vi "Odor_Control_m.vi"() -> ()   [LabVIEW 2014]
uses:
  <vilib>/Utility/file.llb/Read From Spreadsheet File (DBL).vi
  <vilib>/Utility/file.llb/Read From Spreadsheet File (I64).vi
  Image Aquisition - Labview/Image Recorder/experiment state global.vi
  <vilib>/Utility/file.llb/Write To Spreadsheet File (string).vi
panel:
  in  "File with probe valve sequence":path=path "\\\\LABNAS40\\Luis/2016/Physiology_Odor_Responses/Calibration_gwn/gaussian_wn.txt"
  in  "Probe valves from file?":bool
  in  "File with valve sequence":path=path "\\\\LABNAS40\\Luis/2016/Physiology_Odor_Responses/Calibration_gwn/gaussian_wn.txt"
  in  "Valves from file?":bool
  in  "Sync Mode":bool=TRUE
  out "Security Valve \nfor Odor 1":bool
  in  "threshold \nfor odor 1":dbl
  in  "File with signal for odor 2":path=path "\\\\LABNAS40\\Luis/2016/Physiology_Odor_Responses/PL1ol/20170213/step_log_pyramid_w_sigmoid.txt"
  in  "File with signal for odor 1":path=path "\\\\LABNAS40\\Luis/2016/Physiology_Odor_Responses/PL1ol/20170211/Log_pulse_train.txt"
  in  "ODOR 2":bool=TRUE
  in  "ODOR 1":bool
  in  "ODOR 2 FLOW %":dbl(slide) scale=0.0..100.0
  in  "ODOR 1 FLOW %":dbl(slide) scale=0.0..100.0
  in  "ODOR 2":bool=TRUE
  in  "ODOR 1":bool
  in  "TOLERANCE \nFOR CLOSING \nPROBE VALVE":dbl=0.5
  in  "MODE SELECTOR":string(combo)="MANUAL"
  out "Path":path=path "D:/Luis/2017/0212/2118"
  in  "8":bool
  in  "7":bool
  in  "6":bool
  in  "5":bool
  in  "4":bool
  in  "3":bool
  in  "2":bool
  in  "1":bool
  in  "Start Recording":bool
  in  "extra label:":string="Calibration_S3"
  in  "Save To:":path=path "D:/Luis"
  in  "CLEAR stored data":bool
  in  "Select signal to plot":T1(ring)=enum."odor 2 flow rate"
  out "XY Graph":T2(graph)
  in  "Air Flow Rate \n(L/min)":dbl
  in  "odor 2 between experiments":dbl
  in  "odor 2 signal parameters":T3={"temporal ramp type"=enum."Sine", "period(s)"=20.0, "high limit"=0.0, "low limit"=0.0, "duty cycle (sq wave)"=50.0} {"low limit" format="%#_6p"}
  in  "odor 1 between experiments":dbl
  in  "Sync Signal To \nImage Aquisition":bool=TRUE
  in  "ENABLE MFCs":bool
  in  "Restart Signal":bool
  in  "odor 1 signal parameters":T3={"temporal ramp type"=enum."Triangle", "period(s)"=20.0, "high limit"=100.0, "low limit"=10.0, "duty cycle (sq wave)"=50.0} {"low limit" format="%#_6p"}
  in  "update period (ms)":u32=50
  in  "?":bool
  # "NOTE: Always start with Start Recording OFF, don't turn OFF while running"
  # "Manual Stop"
  # "VALVE CONTROL"
  # "MANUAL"
  # "FROM FILE"
  # "VALVE FROM FILE CONTROL"
  # "PREDEFINED WAVEFORM"
  # "PARAMETERS FOR BACKWASH PREVENTION"
  # "Currently the security valve for \nodor 1 is not installed so be careful!"
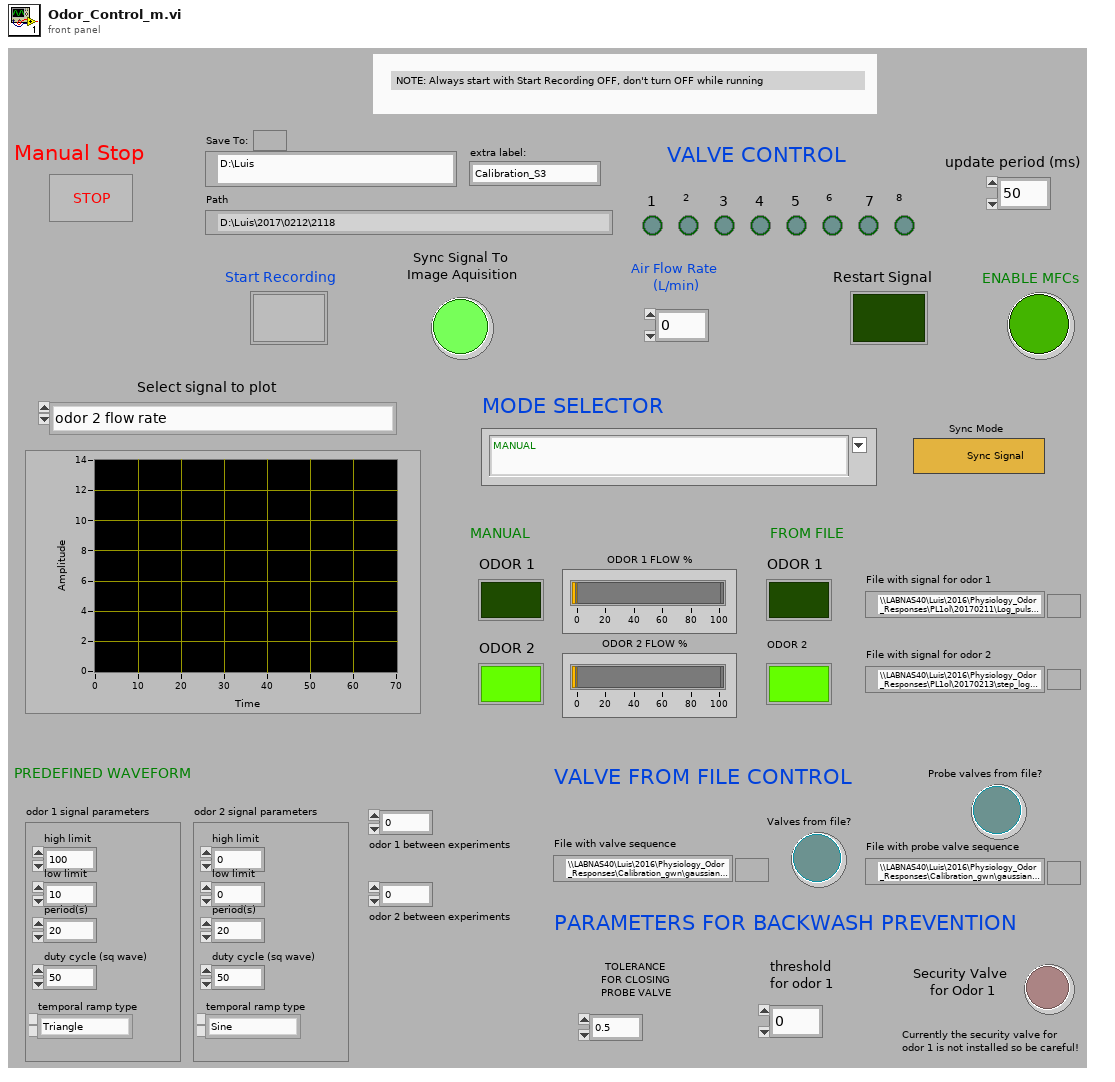
[diagram p1: front panel]
types:
  T1 = enum16{"air setpoint", "air flow rate", "odor 1 set point", "odor 1 flow rate", "odor 2 setpoint", "odor 2 flow rate", "pid reading", "led current", "led voltage", "led setpoint", "led temperature"}
  T2 = cluster{"Value Array":dbl[], "Value Array":dbl[]}
  T3 = cluster{"temporal ramp type":enum16{"Sine", "Triangle", "Sawtooth", "Square", "Exponential"}, "period(s)":dbl, "high limit":dbl, "low limit":dbl, "duty cycle (sq wave)":dbl}
  T4 = cluster{"analog output channels":cluster{"air ao":refnum<k21>, "odor 1 ao":refnum<k21>, "odor 2 ao":refnum<k21>}, "analog input channels":cluster{"air ai":refnum<k21>, "odor 1 ai":refnum<k21>, "odor 2 ai":refnum<k21>, "pid sensor 1 ai":refnum<k21>, "pid sensor 2 ai":refnum<k21>}, "digital control lines":cluster{"air close":refnum<k21>, "air purge":refnum<k21>, "odor 1 close":refnum<k21>, "odor 1 purge":refnum<k21>, "odor 2 close":refnum<k21>, "odor 2 purge":refnum<k21>}}
  T5 = enum16{"Reset Table", "Get Values", "Add Value", "Get Table", "Get Spreadsheet", "set stack writer"}
  T6 = cluster{"experiment started":bool, "experiment ended":bool, "experiment start time":u32}
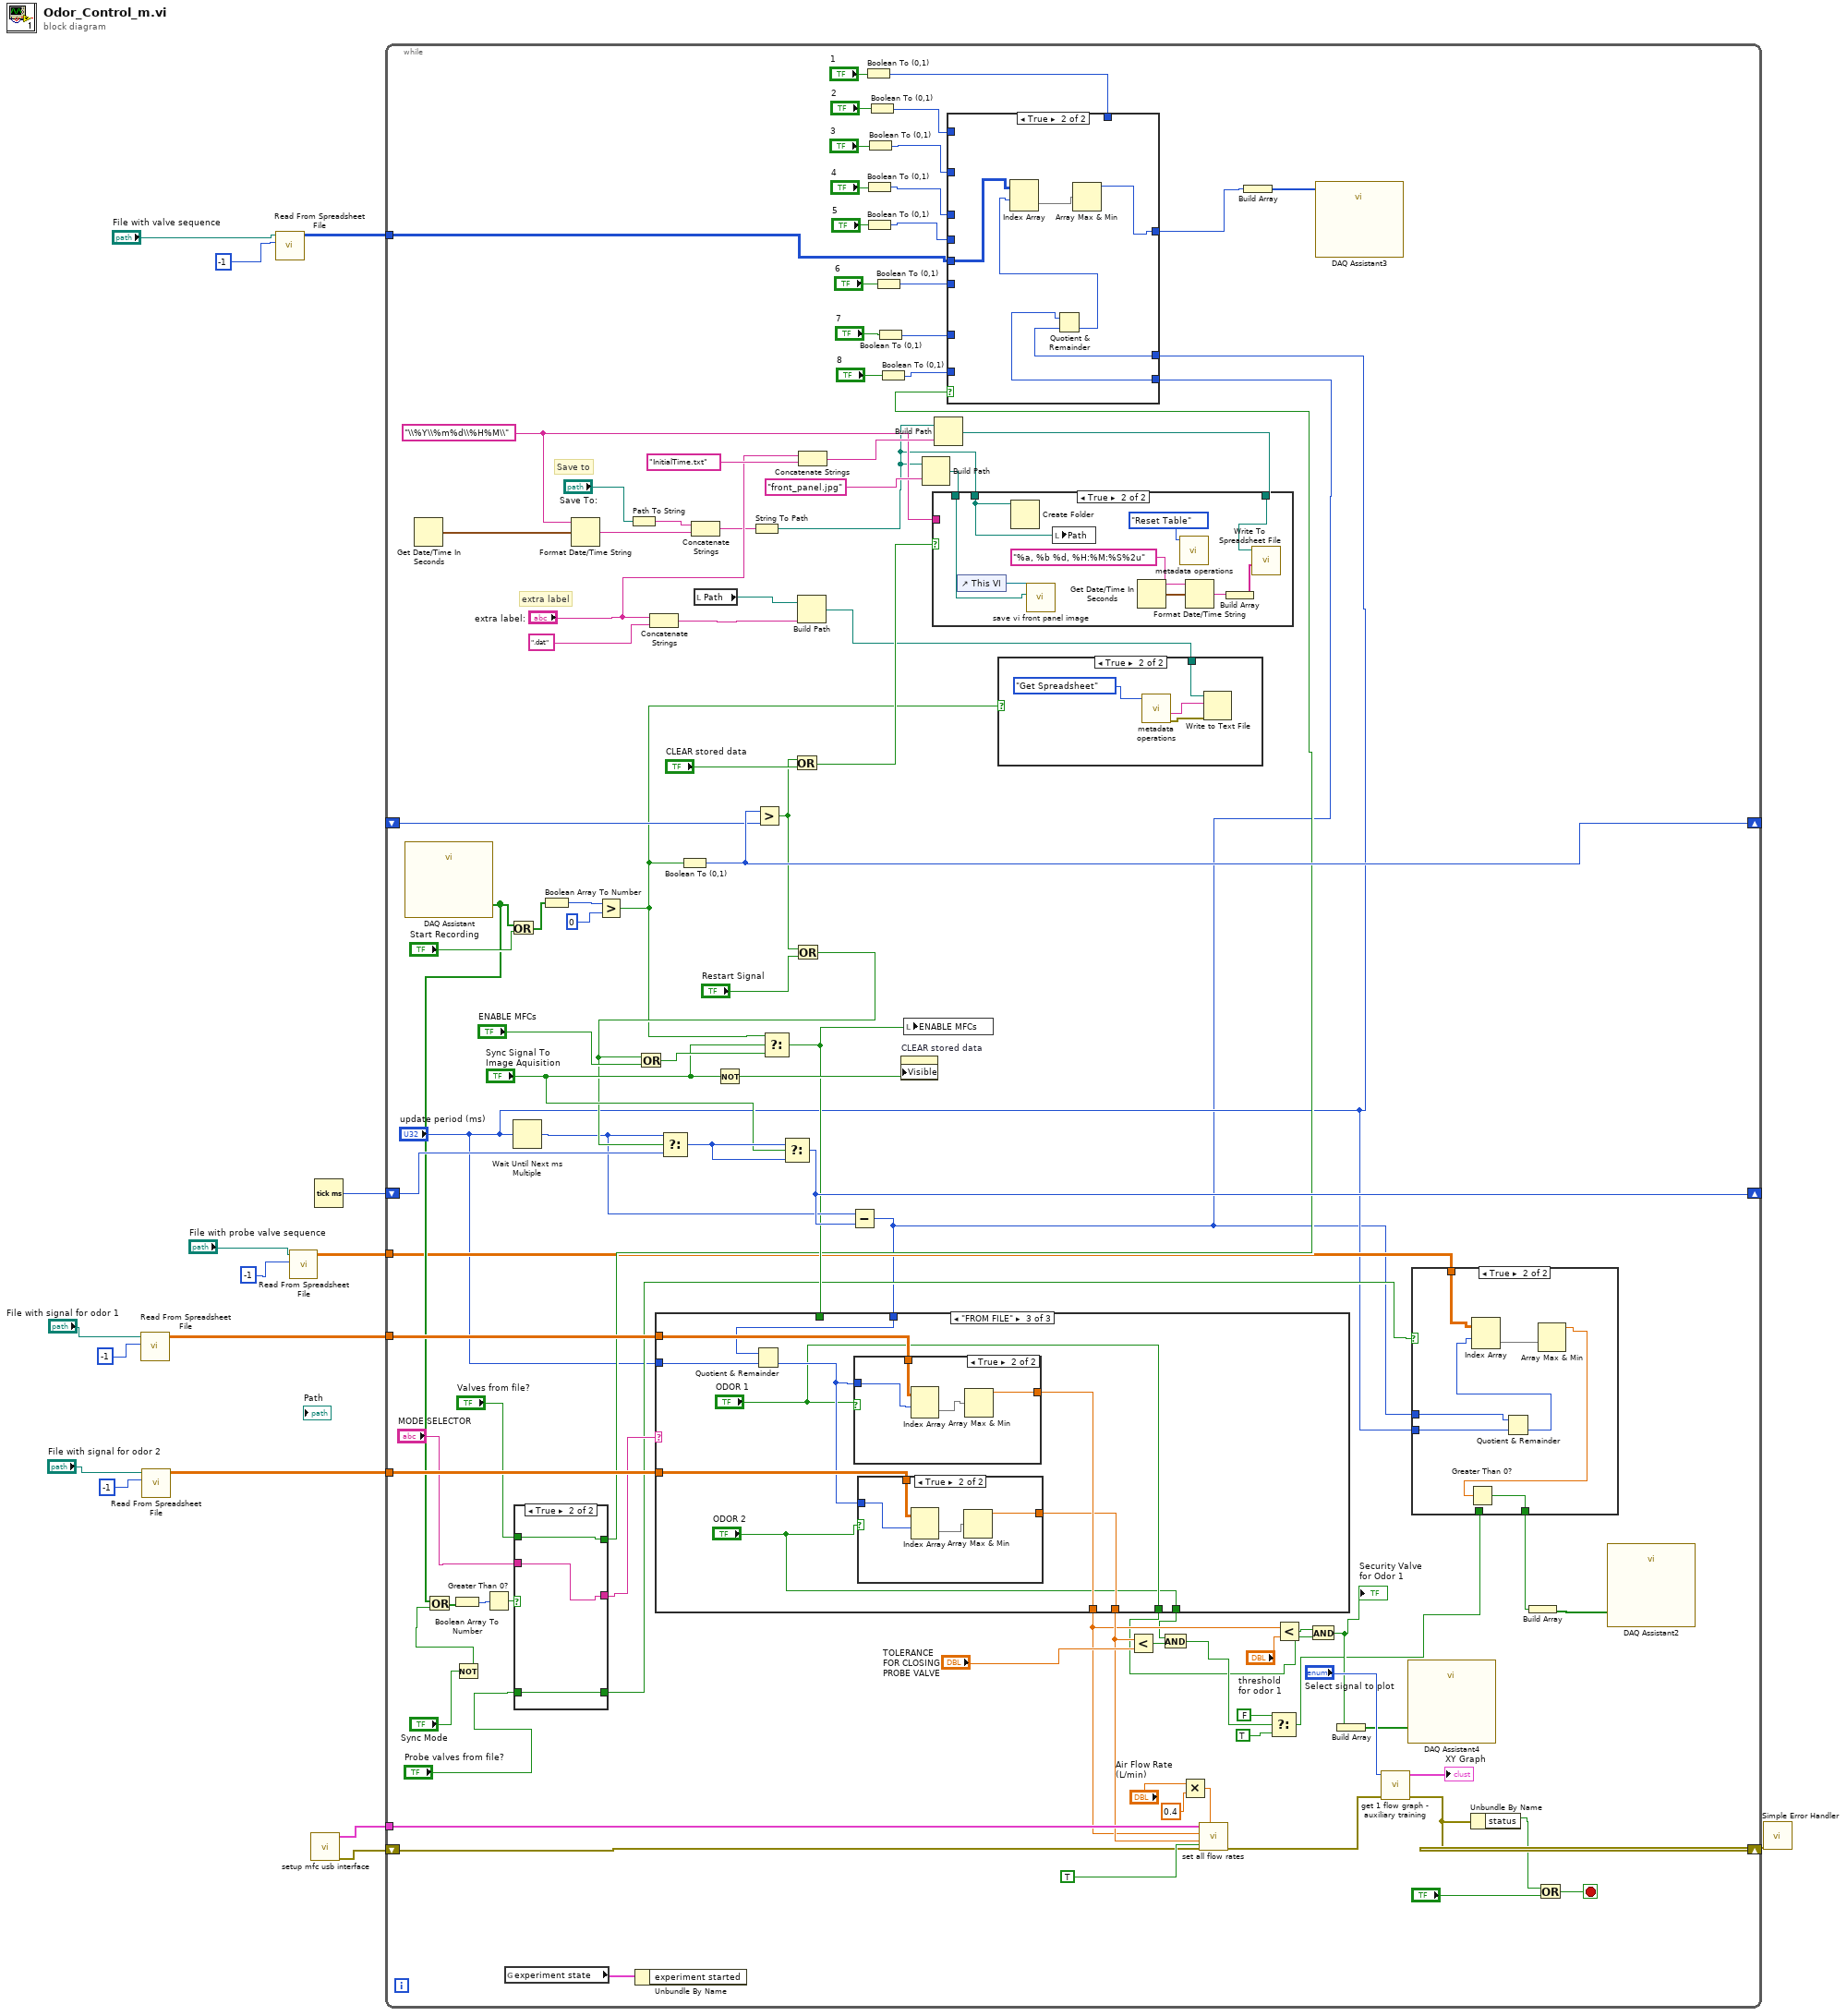
[diagram p0: block diagram]
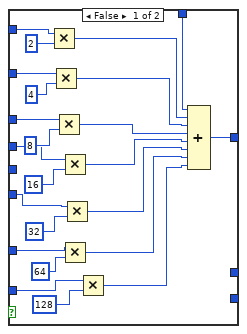
[diagram p3: hidden frame]
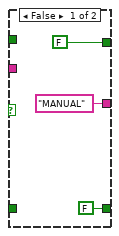
[diagram p4: hidden frame]
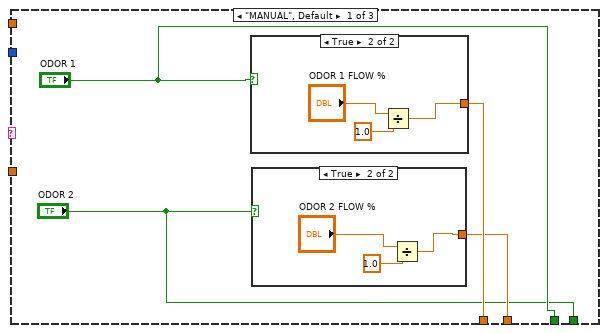
[diagram p5: hidden frame]
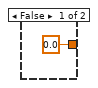
[diagram p6: hidden frame]
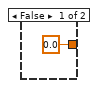
[diagram p7: hidden frame]
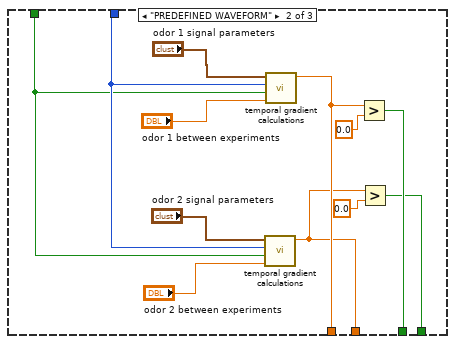
[diagram p8: hidden frame]
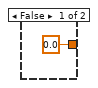
[diagram p9: hidden frame]
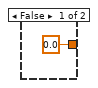
[diagram p10: hidden frame]
diagram:
  n1 = call-poly <vilib>:"Read From Spreadsheet File.vi"("number of rows (all:-1)"=-1, "file path (dialog if empty)"="File with signal for odor 1") -> ("all rows"=w8:dbl[][])  [unwired: 2 in, 7 out]
  n2 = call-poly <vilib>:"Read From Spreadsheet File.vi"("number of rows (all:-1)"=-1, "file path (dialog if empty)"="File with signal for odor 2") -> ("all rows"=w7:dbl[][])  [unwired: 2 in, 7 out]
  n3 = call-poly <vilib>:"Read From Spreadsheet File.vi"("number of rows (all:-1)"=-1, "file path (dialog if empty)"="File with valve sequence") -> ("all rows"=w4:i64[][])  [unwired: 2 in, 7 out]
  n4 = call-poly <vilib>:"Read From Spreadsheet File.vi"("number of rows (all:-1)"=-1, "file path (dialog if empty)"="File with probe valve sequence") -> ("all rows"=w1:dbl[][])  [unwired: 2 in, 7 out]
  n5 = call "setup mfc usb interface.vi"() -> ("error out"=w15:errorcluster, "daqmx tasks"=w14:T4)  [unwired: 10 in]
  n6 = Tick Count (ms)() -> (millisecond timer value=w16:u32)
  n7 = while {
    shift-right: [w66] -> w13
    shift-left: w15 -> [w112]
    shift-right: [w117] -> _
    shift-left: w16 -> [w105]
    tunnel: w14 -> [w111]
    shift-right: [w102] -> _
    shift-left: _ -> [w101]
    tunnel: w8 -> [w62]
    tunnel: w7 -> [w61]
    tunnel: w4 -> [w28]
    tunnel: w1 -> [w25]
    stop <- w120 stop-if-true
    w70 = "\\%Y\\%m%d\\%H%M\\" ("time format string (%c)")
    # "extra label"
    # "Save to"
    n8 = call "DAQ Assistant"() -> ("data"=w43:bool[])  [unwired: 17 in, 2 out]
    n9 = Get Date/Time In Seconds() -> (seconds since 1Jan1904=w79:timestamp)
    n10 = Not(x="Sync Mode") -> (.not. x?=w44:bool)
    n11 = Or(x=w43, y=w44) -> (x .or. y?=w42:bool[])
    n12 = Boolean Array To Number(Boolean array=w42) -> (number=w40:u32)
    n13 = Greater Than 0?(x=w40) -> (x > 0?=w41:bool)
    n14 = global read "experiment state global.vi" "experiment state"() -> (w114:T6)
    n15 = Or(x=w43, y="Start Recording") -> (x .or. y?=w94:bool[])
    n16 = Wait Until Next ms Multiple(millisecond multiple="update period (ms)") -> (millisecond timer value=w67:u32)
    n17 = case shown="True" w41 {
      tunnel: ["MANUAL" ("MODE SELECTOR") w163] -> w47
      tunnel: "MODE SELECTOR" -> [_ w163]
      tunnel: [FALSE w162] -> w39
      tunnel: "Valves from file?" -> [_ w162]
      tunnel: "Probe valves from file?" -> [_ w161]
      tunnel: [FALSE ("Probe valves from file?") w161] -> w26
      frame False {
      }
      frame True {
      }
    }
    n18 = Boolean Array To Number(Boolean array=w94) -> (number=w107:u32)
    n19 = Format Date/Time String(time format string (%c)=w70, seconds (now)=w79) -> (date/time string=w76:string)  [unwired: 1 in]
    n20 = Greater?(x=w107, y=u32 0) -> (0:w68:bool)
    n21 = Path To String(path="Save To:") -> (string=w77:string)
    n22 = Unbundle By Name(w114) -> ()  [unwired: 1 out]
    n23 = Concatenate Strings("extra label:", ".dat" ("name or relative path")) -> (w74:string)
    n24 = Boolean To (0,1)(Boolean=w68) -> (0, 1=w102:i16)
    n25 = Concatenate Strings(w77, w76) -> (w75:string)
    n26 = local read "Path"() -> (w69:path)
    n27 = Not(x="Sync Signal To \nImage Aquisition") -> (.not. x?=w108:bool)
    n28 = String To Path(string=w75) -> (path=w65:path)
    n29 = Greater?(x=w102, y=w101) -> (0:w82:bool)
    n30 = Or(x=w82, y="CLEAR stored data") -> (x .or. y?=w99:bool)
    n31 = Or(x=w82, y="Restart Signal") -> (x .or. y?=w83:bool)
    n32 = Or(x=w83, y="ENABLE MFCs") -> (x .or. y?=w116:bool)
    n33 = Select(t=w67, s=w83, f=w105) -> (s? t:f=w104:u32)
    n34 = Select(t=w68, s="Sync Signal To \nImage Aquisition", f=w116) -> (s? t:f=w64:bool)
    n35 = Select(t=w104, s="Sync Signal To \nImage Aquisition", f=w104) -> (s? t:f=w117:u32)
    n36 = Build Path(base path=w69, name or relative path=w74) -> (appended path=w71:path)
    n37 = Concatenate Strings("extra label:", "InitialTime.txt" ("string")) -> (w81:string)
    n38 = Subtract(x=w67, y=w117) -> (x-y=w23:u32)
    n39 = case shown="\"FROM FILE\"" w47 {
      tunnel: w23 -> [_ w183 w194]
      tunnel: w64 -> [_ w182 _]
      tunnel: [w166 w178 w190] -> w57
      tunnel: [w167 w181 w191] -> w55
      tunnel: w62 -> [_ _ w196]
      tunnel: w61 -> [_ _ w195]
      tunnel: "update period (ms)" -> [_ _ w193]
      tunnel: ["ODOR 1" w180 "ODOR 1"] -> w19
      tunnel: ["ODOR 2" w176 "ODOR 2"] -> w53
      frame "MANUAL", Default {
        n40 = case shown="True" "ODOR 1" {
          tunnel: [0.0 ("ODOR 1 FLOW %") w173] -> w167
          frame False {
          }
          frame True {
            n41 = Divide(x="ODOR 1 FLOW %", y=1.0) -> (x/y=w173:dbl)
          }
        }
        n42 = case shown="True" "ODOR 2" {
          tunnel: [0.0 ("ODOR 2 FLOW %") w169] -> w166
          frame False {
          }
          frame True {
            n43 = Divide(x="ODOR 2 FLOW %", y=1.0) -> (x/y=w169:dbl)
          }
        }
      }
      frame "PREDEFINED WAVEFORM" {
        n44 = call "temporal gradient calculations.vi"("grad disabled value"="odor 2 between experiments", "gradient enabled"=w182, "elapsed time (ms)"=w183, "gradient parameters"="odor 2 signal parameters") -> ("value"=w178:dbl)  [unwired: 7 in]
        n45 = call "temporal gradient calculations.vi"("grad disabled value"="odor 1 between experiments", "gradient enabled"=w182, "elapsed time (ms)"=w183, "gradient parameters"="odor 1 signal parameters") -> ("value"=w181:dbl)  [unwired: 7 in]
        n46 = Greater?(x=w181, y=0.0) -> (0:w180:bool)
        n47 = Greater?(x=w178, y=0.0) -> (0:w176:bool)
      }
      frame "FROM FILE" {
        n48 = Quotient & Remainder(x=w194, y=w193) -> (floor(x/y)=w192:u32)  [unwired: 1 out]
        n49 = case shown="True" "ODOR 1" {
          tunnel: w196 -> [_ w206]
          tunnel: w192 -> [_ w205]
          tunnel: [0.0 w203] -> w191
          frame False {
          }
          frame True {
            n50 = Index Array(array=w206, index (row)=w205) -> (element=w204:dbl[])  [unwired: 1 in]
            n51 = Array Max & Min(array=w204) -> (max value=w203:dbl)  [unwired: 3 out]
          }
        }
        n52 = case shown="True" "ODOR 2" {
          tunnel: w195 -> [_ w201]
          tunnel: w192 -> [_ w200]
          tunnel: [0.0 w198] -> w190
          frame False {
          }
          frame True {
            n53 = Index Array(array=w201, index (row)=w200) -> (element=w199:dbl[])  [unwired: 1 in]
            n54 = Array Max & Min(array=w199) -> (max value=w198:dbl)  [unwired: 3 out]
          }
        }
      }
    }
    n55 = Boolean To (0,1)(Boolean="1") -> (0, 1=w36:i16)
    n56 = Boolean To (0,1)(Boolean="4") -> (0, 1=w34:i16)
    n57 = Boolean To (0,1)(Boolean="5") -> (0, 1=w33:i16)
    n58 = Boolean To (0,1)(Boolean="3") -> (0, 1=w35:i16)
    n59 = Boolean To (0,1)(Boolean="2") -> (0, 1=w37:i16)
    n60 = Boolean To (0,1)(Boolean="6") -> (0, 1=w32:i16)
    n61 = Boolean To (0,1)(Boolean="7") -> (0, 1=w31:i16)
    n62 = Boolean To (0,1)(Boolean="8") -> (0, 1=w30:i16)
    n63 = property on="CLEAR stored data" class="Bool"("Visible"=w108) -> ()  [unwired: 2 in, 2 out]
    n64 = local write "ENABLE MFCs"(w64) -> ()
    n65 = Build Path(base path=w65, name or relative path="front_panel.jpg") -> (appended path=w72:path)
    n66 = Build Path(base path=w65, name or relative path=w81) -> (appended path=w96:path)
    n67 = case shown="True" w99 {
      tunnel: w96 -> [_ w218]
      tunnel: w65 -> [_ w211]
      tunnel: w72 -> [_ w213]
      tunnel: w70 -> [_ _]
      frame False {
      }
      frame True {
        n68 = control-ref of="This VI"() -> (w212:refnum<vi>)
        n69 = Create Folder(path (use dialog)=w211) -> ()  [unwired: 2 in, 3 out]
        n70 = call "save vi front panel image.vi"("path to JPEG file"=w213, "This VI"=w212) -> ()  [unwired: 9 in, 1 out]
        n71 = local write "Path"(w211) -> ()
        n72 = Get Date/Time In Seconds() -> (seconds since 1Jan1904=w217:timestamp)
        n73 = call "metadata operations.vi"("Operation"=T5."Reset Table") -> ()  [unwired: 7 in, 4 out]
        n74 = Format Date/Time String(time format string (%c)="%a, %b %d, %H:%M:%S%2u", seconds (now)=w217) -> (date/time string=w215:string)  [unwired: 1 in]
        n75 = Build Array(w215) -> (w214:string[])
        n76 = call-poly <vilib>:"Write To Spreadsheet File.vi"("1D data"=w214, "file path (dialog if empty)"=w218) -> ()  [unwired: 6 in, 1 out]
      }
    }
    n77 = case shown="True" w39 {
      tunnel: w37 -> [w150 _]
      tunnel: w36 -> [w149 _]
      tunnel: w35 -> [w146 _]
      tunnel: w34 -> [w144 _]
      tunnel: w33 -> [w142 _]
      tunnel: w32 -> [w140 _]
      tunnel: w31 -> [w138 _]
      tunnel: w30 -> [w136 _]
      tunnel: [w129 w155] -> w29
      tunnel: w28 -> [_ w157]
      tunnel: w23 -> [_ w154]
      tunnel: "update period (ms)" -> [_ w153]
      frame False {
        n78 = Multiply(x=w150, y=i16 2) -> (x*y=w148:i16)
        n79 = Multiply(x=w146, y=i16 4) -> (x*y=w135:i16)
        n80 = Multiply(x=w144, y=i16 8) -> (x*y=w134:i16)
        n81 = Multiply(x=w142, y=i16 16) -> (x*y=w133:i16)
        n82 = Multiply(x=w138, y=i16 64) -> (x*y=w131:i16)
        n83 = Multiply(x=w140, y=i16 32) -> (x*y=w132:i16)
        n84 = Multiply(x=w136, y=i16 128) -> (x*y=w130:i16)
        n85 = Compound Arithmetic op=ADD(w149, w148, w135, w134, w133, w132, w131, w130) -> (w129:i16)
      }
      frame True {
        n86 = Quotient & Remainder(x=w154, y=w153) -> (floor(x/y)=w152:u32)  [unwired: 1 out]
        n87 = Index Array(array=w157, index (row)=w152) -> (element=w156:i64[])  [unwired: 1 in]
        n88 = Array Max & Min(array=w156) -> (max value=w155:i64)  [unwired: 3 out]
      }
    }
    n89 = case shown="True" w68 {
      tunnel: w71 -> [_ w210]
      frame False {
      }
      frame True {
        n90 = call "metadata operations.vi"("Operation"=T5."Get Spreadsheet") -> ("error out"=w208:errorcluster, "spreadsheet table"=w207:string)  [unwired: 7 in, 2 out]
        n91 = Write to Text File(file (use dialog)=w210, text=w207, error in=w208) -> ()  [unwired: 1 in, 3 out]
      }
    }
    n92 = Less?(x=w57, y="TOLERANCE \nFOR CLOSING \nPROBE VALVE") -> (x < y?=w54:bool)
    n93 = And(x=w53, y=w54) -> (x .and. y?=w22:bool)
    n94 = Multiply(x="Air Flow Rate \n(L/min)", y=0.4) -> (x*y=w58:dbl)
    n95 = call "set all flow rates.vi"("log flow"=TRUE, "air flow rate"=w58, "error in"=w112, "odor 2 flow rate"=w57, "odor 1 flow rate"=w55, "daqmx tasks"=w111) -> ("error out"=w50:errorcluster)  [unwired: 5 in]
    n96 = Build Array(w29) -> (w85:i64[])
    n97 = Select(t=FALSE, s=w22, f=TRUE) -> (s? t:f=w17:bool)
    n98 = Less?(x=w55, y="threshold \nfor odor 1") -> (x < y?=w20:bool)
    n99 = And(x=w20, y=w19) -> (x .and. y?=w21:bool)
    "Security Valve \nfor Odor 1" <- w21
    n100 = call "DAQ Assistant3"("data"=w85) -> ()  [unwired: 17 in, 2 out]
    n101 = Build Array(w21) -> (w48:bool[])
    n102 = call "get 1 flow graph - auxiliary training.vi"("error in"=w50, "data to plot"="Select signal to plot") -> ("error out"=w66:errorcluster, "graph"=→"XY Graph":T2)  [unwired: 8 in]
    n103 = call "DAQ Assistant4"("data"=w48) -> ()  [unwired: 17 in, 2 out]
    n104 = case shown="True" w26 {
      tunnel: w25 -> [_ w128]
      tunnel: "update period (ms)" -> [_ w126]
      tunnel: w23 -> [_ w125]
      tunnel: [w121 w123] -> w18
      tunnel: w17 -> [w121 _]
      frame False {
      }
      frame True {
        n105 = Quotient & Remainder(x=w125, y=w126) -> (floor(x/y)=w122:u32)  [unwired: 1 out]
        n106 = Index Array(array=w128, index (row)=w122) -> (element=w127:dbl[])  [unwired: 1 in]
        n107 = Array Max & Min(array=w127) -> (max value=w124:dbl)  [unwired: 3 out]
        n108 = Greater Than 0?(x=w124) -> (x > 0?=w123:bool)
      }
    }
    n109 = Unbundle By Name(w66) -> ("status"=w118:bool)
    n110 = Build Array(w18) -> (w49:bool[])
    n111 = Or(x=w118, y="?") -> (x .or. y?=w120:bool)
    n112 = call "DAQ Assistant2"("data"=w49) -> ()  [unwired: 17 in, 2 out]
  }
  n113 = call <vilib>:"Simple Error Handler.vi"("error in (no error)"=w13) -> ()  [unwired: 4 in, 5 out]
